vi "Bundle.vi"(7 "Digit Resolution(5½)":T1=enum."5½", 8 "error in (no error)":errorcluster, 9 "Range":dbl, 10 "Function":T2, 11 "DMM Config Msg in":refnum<class "DMM Config Msg.lvclass">) -> (0 "error out":errorcluster, 3 "DMM Config Msg out":refnum<class "DMM Config Msg.lvclass">)   [LabVIEW 2020, in "DMM Msg.lvlib" / "DMM Config Msg.lvclass"]
doc: "Populate the DMM Config Msg."
uses:
  DMM Config Msg.lvclass
  PPL/HDH.Driver.DMM.lvlibp/Controls/Ctl_Function.ctl
  PPL/HDH.Driver.DMM.lvlibp/Controls/Ctl_DigitResolution.ctl
  DMM Config Msg.lvclass/DMM Config Msg.ctl
  PPL/HDH.Driver.DMM.lvlibp
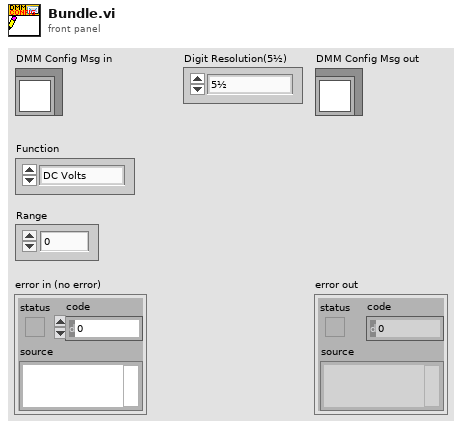
[diagram p1: front panel]
types:
  T1 = typedef "HDH.Driver.DMM.lvlibp/Ctl_DigitResolution.ctl" = enum8{"3½", "4½", "5½", "6½", "7½"}
  T2 = typedef "HDH.Driver.DMM.lvlibp/Ctl_Function.ctl" = enum8{"DC Volts", "AC Volts", "DC Current", "AC Current", "2-wire Resistance", "4-wire Resistance", "Diode", "Frequency", "Period", "AC Volts DC Coupled", "Capacitance", "Inductance", "Temperature"}
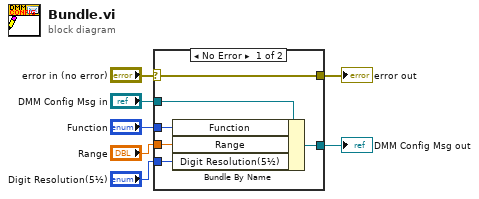
[diagram p0: block diagram]
diagram:
  n1 = case shown="No Error" "error in (no error)" {
    selector: "error in (no error)" -> [w13 w14]
    tunnel: [w13 w14] -> w6
    tunnel: [w11 w15] -> w4
    tunnel: "DMM Config Msg in" -> [w12 w15]
    tunnel: "Function" -> [w10 _]
    tunnel: "Range" -> [w9 _]
    tunnel: "Digit Resolution(5½)" -> [w8 _]
    frame No Error {
      n2 = Bundle By Name(cluster=w12, "Function"=w10, "Range"=w9, "Digit Resolution(5½)"=w8) -> (w11:refnum<class "DMM Config Msg.lvclass">)
    }
    frame Error {
    }
  }
  "error out" <- w6
  "DMM Config Msg out" <- w4
